vi "readSDOU16.vi"() -> ()   [LabVIEW 2018, in "MotorControllerClass.lvclass"]
uses:
  BMS/MotorControllerClass.lvclass
  <vilib>/CANopenLib/CANOPEN.llb/CANopen SDO Create.vi
  <vilib>/CANopenLib/CANOPEN.llb/CANopen SDO Read [U16].vi
  <vilib>/CANopenLib/CANOPEN.llb/CANopen SDO Close.vi
panel:
  out "MotorControllerClass out":refnum<class "MotorControllerClass.lvclass">
  in  "MotorControllerClass in":refnum<class "MotorControllerClass.lvclass">
  out "completion code":u32 format="%.0x"
  out "interface object out":refnum<k20>
  in  "interface object in":refnum<k20>
  in  "objectIndex":u16 format="%x"
  in  "subIndex":u8
  out "output":u16
  out "error out":errorcluster
  in  "error in (no error)":errorcluster
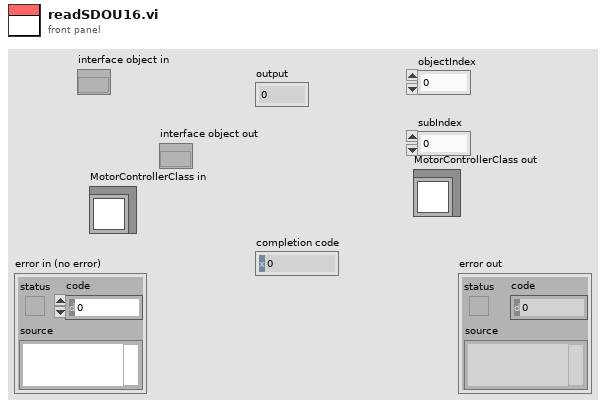
[diagram p1: front panel]
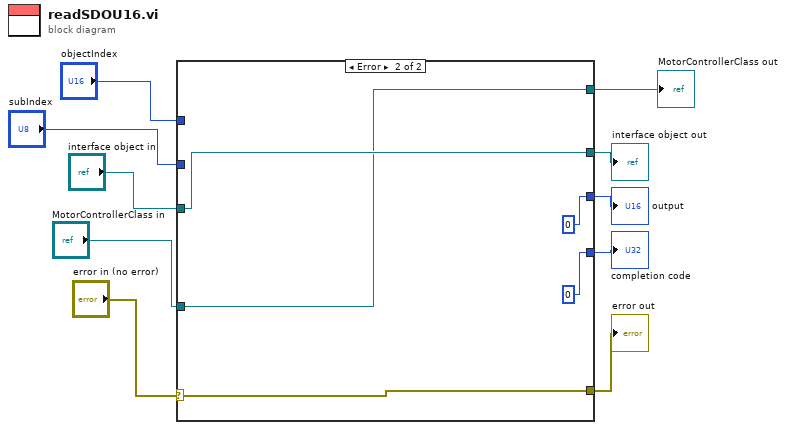
[diagram p0: block diagram]
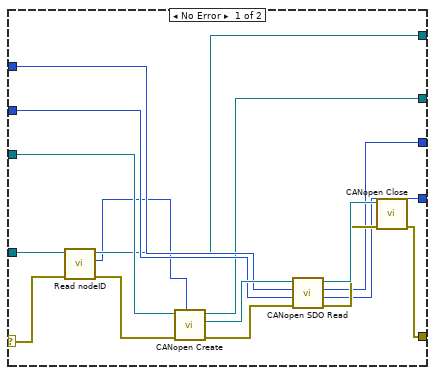
[diagram p2: hidden frame]
diagram:
  n1 = case shown="Error" "error in (no error)" {
    selector: "error in (no error)" -> [w15 w31]
    tunnel: [w19 w31] -> w4
    tunnel: "subIndex" -> [w22 _]
    tunnel: "objectIndex" -> [w21 _]
    tunnel: "interface object in" -> [w20 w30]
    tunnel: [w18 w30] -> w7
    tunnel: [w17 u32 0 ("completion code")] -> w6
    tunnel: [w16 u16 0 ("U16 data")] -> w3
    tunnel: "MotorControllerClass in" -> [w13 w27]
    tunnel: [w12 w27] -> w1
    frame No Error {
      n2 = call-dynamic "Read nodeID.vi"("error in (no error)"=w15, "MotorControllerClass in"=w13) -> ("error out"=w14:errorcluster, "nodeID"=w11:u8, "MotorControllerClass out"=w12:refnum<class "MotorControllerClass.lvclass">)  [unwired: 7 in]
      n3 = call-poly <vilib>:"CANopen Create.vi"("node-ID"=w11, "error in (no error)"=w14, "interface object in"=w20) -> ("error out"=w26:errorcluster, "SDO object out"=w25:refnum<k20>, "interface object out"=w18:refnum<k20>)  [unwired: 6 in]
      n4 = call-poly <vilib>:"CANopen SDO Read.vi"("error in (no error)"=w26, "object sub-index (0)"=w22, "object index"=w21, "SDO object in"=w25) -> ("error out"=w23:errorcluster, "completion code"=w17:u32, "U16 data"=w16:u16, "SDO object out"=w24:refnum<k20>)  [unwired: 4 in]
      n5 = call-poly <vilib>:"CANopen Close.vi"("error in (no error)"=w23, "SDO object in"=w24) -> ("error out"=w19:errorcluster)  [unwired: 9 in]
    }
    frame Error {
    }
  }
  "error out" <- w4
  "output" <- w3
  "interface object out" <- w7
  "completion code" <- w6
  "MotorControllerClass out" <- w1
